vi "getReadFile.vi"(1 "Folder Path":path) -> (0 "error out":errorcluster)   [LabVIEW 2013]
uses:
  Globals/measurementGlobal.vi
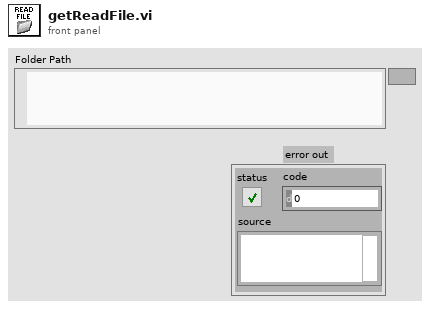
[diagram p1: front panel]
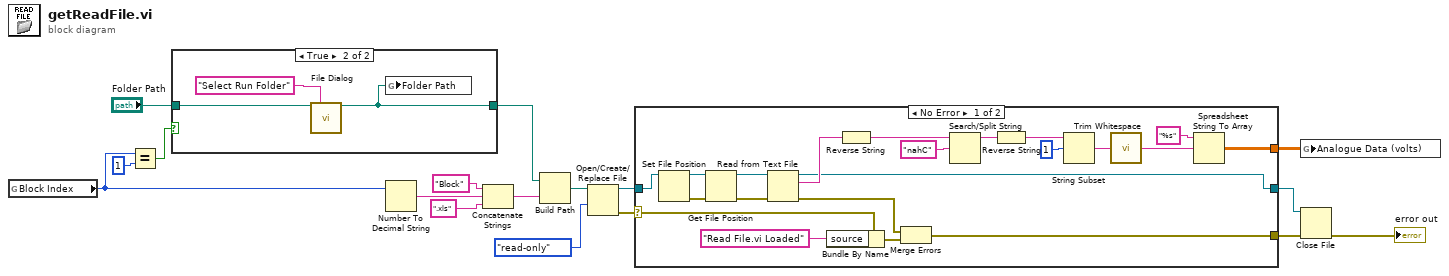
[diagram p0: block diagram]
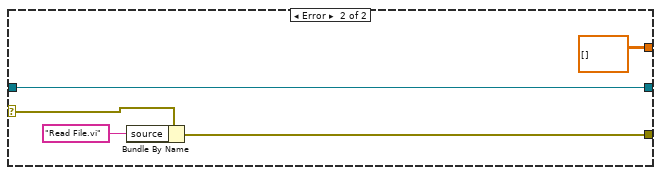
[diagram p3: hidden frame]
diagram:
  n1 = global read "measurementGlobal.vi" "Block Index"() -> (w4:i32)
  n2 = Equal?(x=w4, y=1) -> (x = y?=w2:bool)
  n3 = case shown="True" w2 {
    tunnel: "Folder Path" -> [w18 w21]
    tunnel: [w18 w19] -> w10
    frame False {
    }
    frame True {
      n4 = call "File Dialog"("start path"=w21, "prompt"="Select Run Folder") -> ("selected path"=w19:path)  [unwired: 10 in, 3 out]
      n5 = global write "measurementGlobal.vi" "Folder Path"(w19) -> ()
    }
  }
  n6 = Number To Decimal String(number=w4) -> (decimal integer string=w7:string)  [unwired: 1 in]
  n7 = Concatenate Strings("Block" ("name or relative path"), w7, ".xls" ("name or relative path")) -> (w5:string)
  n8 = Build Path(base path=w10, name or relative path=w5) -> (appended path=w9:path)
  n9 = Open/Create/Replace File(file path (use dialog)=w9, access (0:read/write)=enum16{"read/write", "read-only", "write-only"}."read-only") -> (refnum out=w16:refnum<file>, error out=w12:errorcluster)  [unwired: 4 in, 1 out]
  n10 = case shown="No Error" w12 {
    selector: w12 -> [w28 w44]
    tunnel: w16 -> [w42 w47]
    tunnel: [w22 w47] -> w15
    tunnel: [w25 w43] -> w14
    tunnel: [w24 dbl[][] []] -> w11
    frame No Error {
      n11 = Set File Position(refnum=w42) -> (refnum out=w41:refnum<file>, error out=w40:errorcluster)  [unwired: 3 in]
      n12 = Get File Position(4:w40, 7:w41) -> (0:w39:errorcluster, 3:w38:refnum<file>)  [unwired: 1 out]
      n13 = Read from Text File(file (use dialog)=w38, error in=w39) -> (refnum out=w22:refnum<file>, text=w37:string, error out=w23:errorcluster)  [unwired: 2 in, 1 out]
      n14 = Bundle By Name(cluster=w28, "source"="Read File.vi Loaded") -> (w26:errorcluster)
      n15 = Reverse String(1:w37) -> (0:w36:string)
      n16 = Merge Errors(w23, w26) -> (w25:errorcluster)
      n17 = Search/Split String(string=w36, search string/char (-)="nahC") -> (substring before match=w34:string)  [unwired: 1 in, 2 out]
      n18 = Reverse String(1:w34) -> (0:w33:string)
      n19 = String Subset(string=w33, offset (0)=1) -> (substring=w30:string)  [unwired: 1 in]
      n20 = call <vilib>:"Trim Whitespace.vi"("string"=w30) -> ("trimmed string"=w29:string)  [unwired: 1 in]
      n21 = Spreadsheet String To Array(format string="%s", spreadsheet string=w29) -> (array=w24:dbl[][])  [unwired: 2 in]
    }
    frame Error {
      n22 = Bundle By Name(cluster=w44, "source"="Read File.vi") -> (w43:errorcluster)
    }
  }
  n23 = global write "measurementGlobal.vi" "Analogue Data (volts)"(w11) -> ()
  n24 = Close File(refnum=w15, error in=w14) -> (error out=→"error out":errorcluster)  [unwired: 1 out]
